vi "Schedule Poll.vi"(8 "error in":errorcluster, 11 "Instruments in":refnum<class "Instruments.lvclass">) -> (0 "error out":errorcluster, 3 "Instruments out":refnum<class "Instruments.lvclass">)   [LabVIEW 2023, in "Instruments.lvlib" / "Instruments.lvclass"]
doc: "Schedule Measurement Polling - This is disabled when an error is present. This prevents filling a failed to launch machine's message queue which causes severe damage to the behavior of the system."
uses:
  Library/Instruments.lvclass
  C:/Users/Public/Documents/Development/builds/Engine/Engine.lvlibp/Project/Engine.lvclass
  Instruments Messages/Measure Msg/Measure Msg.lvclass
  C:/Users/Public/Documents/Development/builds/Engine/Actor Framework.lvlibp/1abvi3w/vi.lib/ActorFramework/Message/Message.lvclass
  Library/Instruments.lvclass/Instruments.ctl
  Private/Accessors/Read Poll(ms).vi
  builds/Engine/Engine.lvlibp/Accessors/Read Self Q.vi
  builds/Engine/Actor Framework.lvlibp/1abvi3w/vi.lib/ActorFramework/Message Enqueuer/Message Enqueuer.lvclass
  builds/Engine/Actor Framework.lvlibp
  builds/Engine/Engine.lvlibp/Project/Engine.lvclass
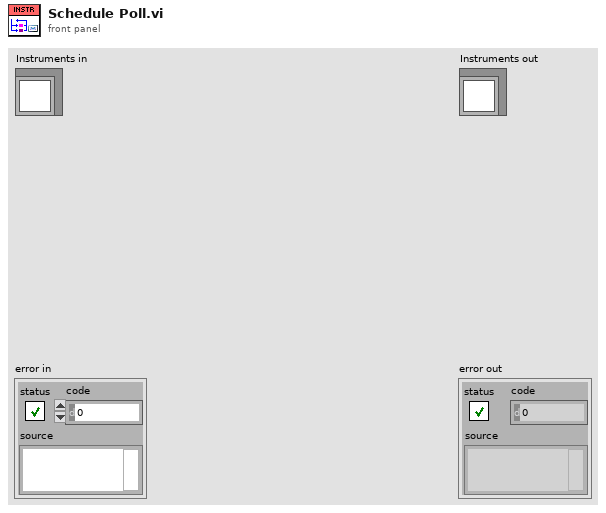
[diagram p1: front panel]
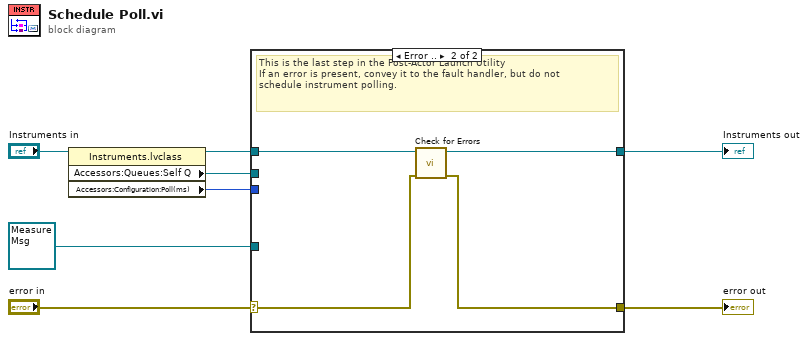
[diagram p0: block diagram]
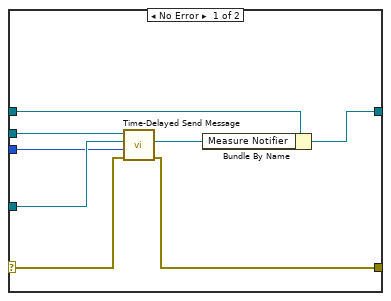
[diagram p2: hidden frame]
diagram:
  n1 = property class="Instruments.lvclass"(reference="Instruments in") -> (reference out=w5:refnum<class "Instruments.lvclass">, "Accessors:Queues:Self Q"=w6:refnum<class "Message Enqueuer.lvclass">, "Accessors:Configuration:Poll(ms)"=w3:u32)  [unwired: 1 in, 1 out]
  n2 = case shown="Error .." "error in" {
    selector: "error in" -> [w10 w18]
    tunnel: refnum<class "Measure Msg.lvclass"> refnum ("Instruments.lvlib:Measure Msg.lvclass") -> [w16 _]
    tunnel: w6 -> [w15 _]
    tunnel: w5 -> [w14 w20]
    tunnel: [w13 w19] -> w4
    tunnel: w3 -> [w11 _]
    tunnel: [w9 w17] -> w1
    frame No Error {
      n3 = call "Time-Delayed Send Message.vi"("error in (no error)"=w10, "Milliseconds To Wait"=w11, "Message"=w16, "Message Enqueuer"=w15) -> ("error out"=w9:errorcluster, "Delivery Notifier"=w12:refnum<notifier>)  [unwired: 6 in]
      n4 = Bundle By Name(cluster=w14, "Measure Notifier"=w12) -> (w13:refnum<class "Instruments.lvclass">)
    }
    frame Error {
      # "This is the last step in the Post-Actor Launch Utility\nIf an error is present, convey it to the fault handler, but do not \nschedule instrument polling."
      n5 = call "Check for Errors.vi"("error in"=w18, "Engine in"=w20) -> ("error out"=w17:errorcluster, "Engine out"=w19:refnum<class "Instruments.lvclass">)  [unwired: 8 in]
    }
  }
  "error out" <- w1
  "Instruments out" <- w4
